vi "Transform Numeric Input to Double.vi"(10 "LSS String Value as Variant":variant, 11 "Value from Control":variant) -> (2 "Expected":dbl, 3 "Control":dbl)   [LabVIEW 2019, in "LSS.lvlib"]
doc: "Transforms the two inputs to doubles that can be properly compared."
uses:
  LSS.lvlib
  <vilib>/Utility/Data Type/Type Definitions/Data Type.ctl
  <vilib>/Utility/Data Type/NI_Data Type.lvlib
panel:
  out "Type":T1
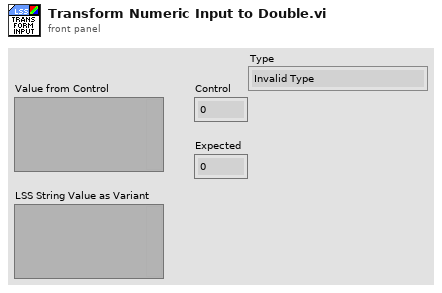
[diagram p1: front panel]
types:
  T1 = typedef "NI_Data Type.lvlib/Data Type.ctl" = enum8{"Invalid Type", "Void", "I8", "I16", "I32", "I64", "U8", "U16", "U32", "U64", "Single Float", "Double Float", "Extended Float", "Single Complex", "Double Complex", "Extended Complex", "Enum U8", "Enum U16", "Enum U32", "Enum U64", "Single Float With Unit", "Double Float With Unit", "Extended Float With Unit", "Single Complex with Unit", "Double Complex with Unit", "Extended Complex with Unit", "Boolean", "String", "Path", "Picture", "Tag", "Array", "Cluster", "Variant", "LV Variant", "Waveform", "Timestamp", "Digital Waveform", "Digital Data", "ExpressData", "Refnum", "External Data", "VI", "Poly VI", "LabVIEW Class Instance", "Fixed Point", "Set Collection", "Map Collection"}
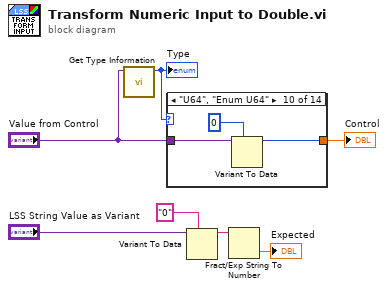
[diagram p0: block diagram]
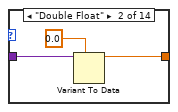
[diagram p3: hidden frame]
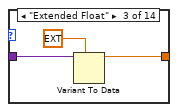
[diagram p4: hidden frame]
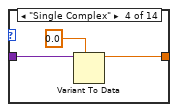
[diagram p5: hidden frame]
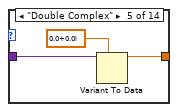
[diagram p6: hidden frame]
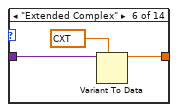
[diagram p7: hidden frame]
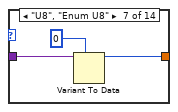
[diagram p8: hidden frame]
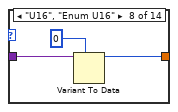
[diagram p9: hidden frame]
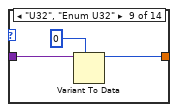
[diagram p10: hidden frame]
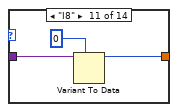
[diagram p11: hidden frame]
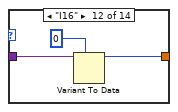
[diagram p12: hidden frame]
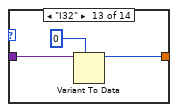
[diagram p13: hidden frame]
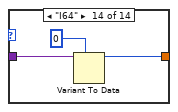
[diagram p14: hidden frame]
diagram:
  n1 = call <vilib>:"Get Type Information.vi"("variant"="Value from Control") -> ("type"=w3:T1)  [unwired: 6 in, 4 out]
  "Type" <- w3
  n2 = case shown="\"U64\", \"Enum U64\"" w3 {
    tunnel: "Value from Control" -> [_ w9 w12 w15 w18 w21 w24 w27 w30 w33 w36 w39 w42 w45]
    tunnel: [_ w8 w11 w14 w17 w20 w23 w26 w29 w32 w35 w38 w41 w44] -> w2
    frame "Invalid Type", Default {
    }
    frame "Double Float" {
      n3 = Variant To Data(type=0.0 ("x"), Variant=w9) -> (data=w8:dbl)  [unwired: 1 in, 1 out]
    }
    frame "Extended Float" {
      n4 = Variant To Data(type=ext 0.0 ("x"), Variant=w12) -> (data=w11:ext)  [unwired: 1 in, 1 out]
    }
    frame "Single Complex" {
      n5 = Variant To Data(type=sgl 0.0 ("x"), Variant=w15) -> (data=w14:sgl)  [unwired: 1 in, 1 out]
    }
    frame "Double Complex" {
      n6 = Variant To Data(type=cdb 0.0+0.0i ("x"), Variant=w18) -> (data=w17:cdb)  [unwired: 1 in, 1 out]
    }
    frame "Extended Complex" {
      n7 = Variant To Data(type=cxt 0.0+0.0i ("x"), Variant=w21) -> (data=w20:cxt)  [unwired: 1 in, 1 out]
    }
    frame "U8", "Enum U8" {
      n8 = Variant To Data(type=u8 0 ("x"), Variant=w24) -> (data=w23:u8)  [unwired: 1 in, 1 out]
    }
    frame "U16", "Enum U16" {
      n9 = Variant To Data(type=u16 0 ("x"), Variant=w27) -> (data=w26:u16)  [unwired: 1 in, 1 out]
    }
    frame "U32", "Enum U32" {
      n10 = Variant To Data(type=u32 0 ("x"), Variant=w30) -> (data=w29:u32)  [unwired: 1 in, 1 out]
    }
    frame "U64", "Enum U64" {
      n11 = Variant To Data(type=u64 0 ("x"), Variant=w33) -> (data=w32:u64)  [unwired: 1 in, 1 out]
    }
    frame "I8" {
      n12 = Variant To Data(type=i8 0 ("x"), Variant=w36) -> (data=w35:i8)  [unwired: 1 in, 1 out]
    }
    frame "I16" {
      n13 = Variant To Data(type=i16 0 ("x"), Variant=w39) -> (data=w38:i16)  [unwired: 1 in, 1 out]
    }
    frame "I32" {
      n14 = Variant To Data(type=0 ("x"), Variant=w42) -> (data=w41:i32)  [unwired: 1 in, 1 out]
    }
    frame "I64" {
      n15 = Variant To Data(type=i64 0 ("x"), Variant=w45) -> (data=w44:i64)  [unwired: 1 in, 1 out]
    }
  }
  "Control" <- w2
  n16 = Variant To Data(type="0" ("Numeric 2"), Variant="LSS String Value as Variant") -> (data=w5:string)  [unwired: 1 in, 1 out]
  n17 = Fract/Exp String To Number(string=w5) -> (number=→"Expected":dbl)  [unwired: 3 in, 1 out]
